vi "Error站_Run.vi"(8 "error in":errorcluster, 9 "Function":T1, 10 "Mode":T2, 11 "ref in":T3) -> (0 "error out":errorcluster, 3 "ref out":T3)   [LabVIEW 2015]
doc: "Use this template to build a VI to use as a subVI."
panel:
  out "Timed out":bool
  in  "ms timeout (-1)":i32=-1
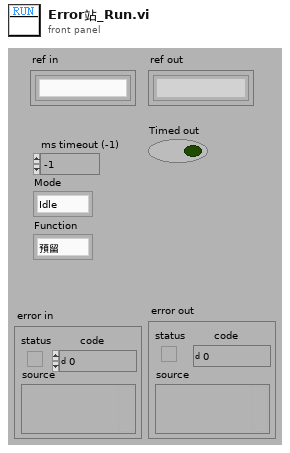
[diagram p1: front panel]
types:
  T1 = typedef "Error站_Function.ctl" = enum8{"預留"}
  T2 = typedef "Error站_Mode.ctl" = enum8{"Idle", "Run", "Pause", "Err"}
  T3 = typedef "Error站_ref.ctl" = refnum<k1>
  T4 = enum16{"OpenReference", "CloseReference", "Get Data", "Set Data", "Set Flag"}
  T5 = typedef "Semaphore RefNum" = refnum<k1>
  T6 = typedef "Error站_Data.ctl" = cluster{"GUI":refnum<vi>, "Ready":bool, "Mode":T2, "Function":T1, "Porcedure in":u8, "Time Delay":cluster{"Time Out":dbl, "氣壓缸延遲":dbl, "3":dbl, "4":dbl, "5":dbl, "6":dbl, "7":dbl, "8":dbl, "9":dbl, "10":dbl}, "空跑流程":bool, "異常處理":cluster{"Retry":bool, "Reset":bool, "Skip":bool}, "Message Array":i32[]}
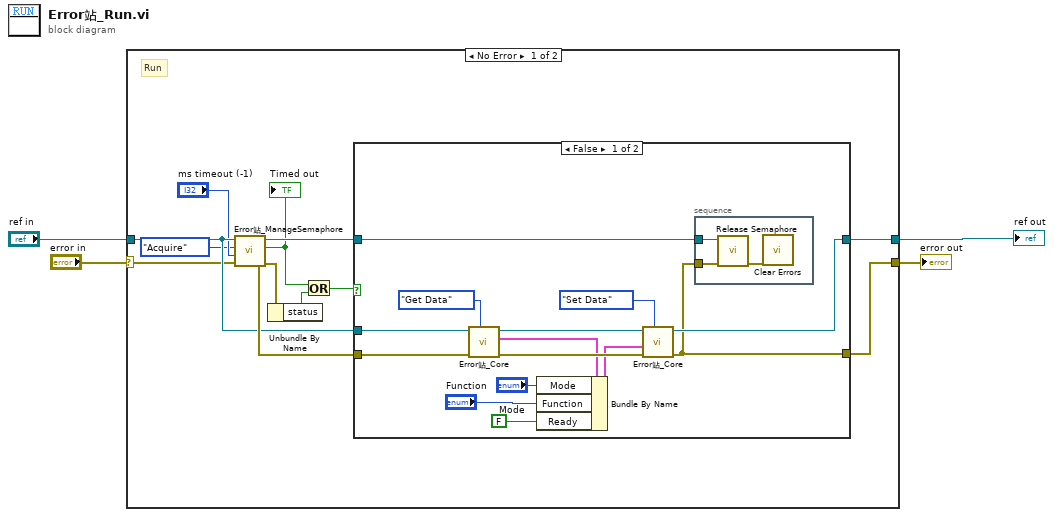
[diagram p0: block diagram]
diagram:
  n1 = case shown="No Error" "error in" {
    selector: "error in" -> [w6 w35]
    tunnel: [w10 w35] -> w3
    tunnel: "ref in" -> [w11 w34]
    tunnel: [w12 w34] -> w1
    frame No Error {
      # "Run"
      n2 = call "Error站_ManageSemaphore.vi"("error in (no error)"=w6, "ms timeout (-1)"="ms timeout (-1)", "Method (Acquire)"=enum8{"Acquire", "Destroy"}."Acquire", "ref"=w11) -> ("error out"=w15:errorcluster, "Timed out"=w7:bool, "semaphore out"=w13:T5)  [unwired: 1 in]
      "Timed out" <- w7
      n3 = Unbundle By Name(w15) -> ("status"=w8:bool)
      n4 = Or(x=w7, y=w8) -> (x .or. y?=w14:bool)
      n5 = case shown="False" w14 {
        tunnel: [w27 w32] -> w12
        tunnel: w13 -> [w28 _]
        tunnel: w15 -> [w25 w33]
        tunnel: [w26 w33] -> w10
        tunnel: w11 -> [w24 w32]
        frame False {
          n6 = call "Error站_Core.vi"("Function"=T4."Get Data", "ref in"=w24) -> ("Data out"=w22:T6, "ref out"=w23:T3)  [unwired: 6 in, 2 out]
          n7 = Bundle By Name(cluster=w22, "Mode"="Mode", "Function"="Function", "Ready"=FALSE) -> (w18:T6)
          n8 = call "Error站_Core.vi"("Function"=T4."Set Data", "error in"=w25, "Data in"=w18, "ref in"=w23) -> ("error out"=w26:errorcluster, "ref out"=w27:T3)  [unwired: 4 in, 2 out]
          n9 = stacked-sequence {
            tunnel: w28 -> [w31]
            tunnel: w26 -> [w29]
            frame #0 {
              n10 = call <vilib>:"Release Semaphore.vi"("error in (no error)"=w29, "semaphore"=w31) -> ("error out"=w30:errorcluster)  [unwired: 4 in, 1 out]
              n11 = call <vilib>:"Clear Errors.vi"("error in (no error)"=w30) -> ()  [unwired: 5 in, 2 out]
            }
          }
        }
        frame True {
        }
      }
    }
    frame Error {
    }
  }
  "error out" <- w3
  "ref out" <- w1
